vi "Dax_RadValsBP2.vi"(10 "Num Channels":i32=5, 11 "Daxsonics":refnum<visa-resource-name>="Daxsonics") -> (0 "Dax Values":cluster{"Freq":i32, "Amp":i32, "Gain":i32}, 1 "Freq (MHz)":u16=5, 2 "Amp (V)":u16, 3 "Gains":u16[](array[numeric]))   [LabVIEW 2022 SP3]
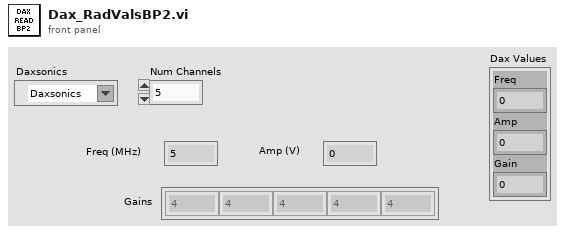
[diagram p1: front panel]
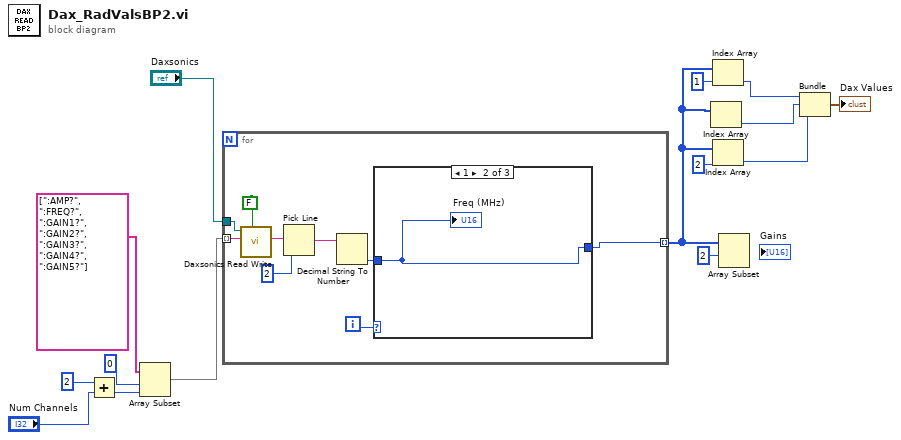
[diagram p0: block diagram]
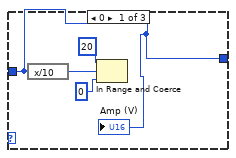
[diagram p2: hidden frame]
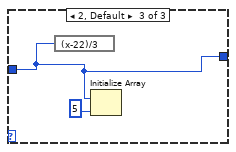
[diagram p3: hidden frame]
diagram:
  n1 = Add(x=2, y="Num Channels") -> (x+y=w9:i32)
  n2 = Array Subset(array=string[] [":AMP?", ":FREQ?", ":GAIN1?", ":GAIN2?", ":GAIN3?", ":GAIN4?", ":GAIN5?"], index=0, length=w9) -> (w12:string[])
  n3 = for {
    tunnel: w12 -> [w22] mode=indexing
    tunnel: "Daxsonics" -> [w18]
    tunnel: [w16] -> w7 mode=indexing
    i -> [w24]
    n4 = call "Daxsonics Read Write.vi"("Daxsonics Name"=FALSE ("Enable Termination\nChar (T)"), "write buffer"=w22, "VISA resource name"=w18) -> ("read buffer"=w21:string)  [unwired: 6 in, 2 out]
    n5 = Pick Line(multi-line string=w21, line index=2) -> (output string=w20:string)  [unwired: 1 in]
    n6 = Decimal String To Number(string=w20) -> (number=w23:i32)  [unwired: 2 in, 1 out]
    n7 = case shown="1" w24 {
      tunnel: w23 -> [w25 w29 w30]
      tunnel: [w25 w29 w30] -> w16
      frame 0 {
        n8 = expression code="x/10"(w25) -> (w28:i32)
        n9 = In Range and Coerce(upper limit=20, x=w28, lower limit=0) -> ()  [unwired: 2 out]
        "Amp (V)" <- w25
      }
      frame 1 {
        "Freq (MHz)" <- w29
      }
      frame 2, Default {
        n10 = expression code="(x-22)/3"(w30) -> ()  [unwired: 1 out]
        n11 = Initialize Array(w30, 5 ("dimension size")) -> ()  [unwired: 1 out]
      }
    }
  }
  n12 = Index Array(array=w7) -> (element=w5:i32)  [unwired: 1 in]
  n13 = Index Array(array=w7, index=1) -> (element=w6:i32)
  n14 = Index Array(array=w7, index=2) -> (element=w4:i32)
  n15 = Array Subset(array=w7, index=2) -> ()  [unwired: 1 in, 1 out]
  n16 = Bundle(w6, w5, w4) -> (→"Dax Values":cluster{i32, i32, i32})  [unwired: 1 in]
